vi "Init AI Resources.vi"(8 "error in (no error)":errorcluster, 11 "Session in":refnum<class "Session.lvclass">) -> (0 "error out":errorcluster, 3 "Session out":refnum<class "Session.lvclass">)   [LabVIEW 2024, in "CTI.lvlib" / "Session.lvclass"]
uses:
  Session.lvclass
  ADC Number.ctl
  AI/AI.lvclass
  Session.lvclass/Session.ctl
  CTI.lvlib
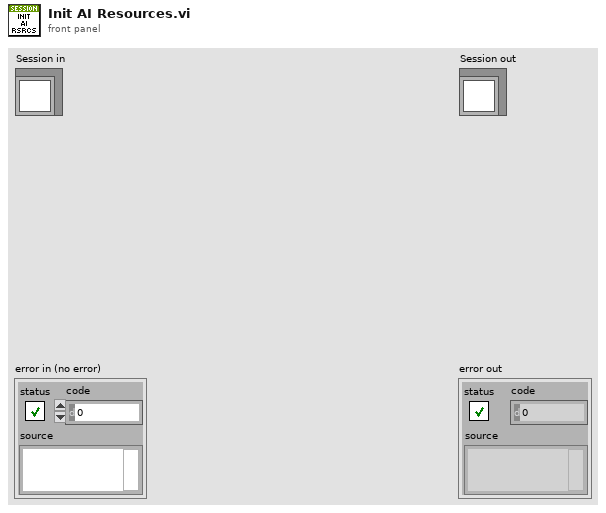
[diagram p1: front panel]
types:
  T1 = typedef "CTI.lvlib/ADC Number.ctl" = i8
  T2 = typedef "CTI.lvlib/Available AI.ctl" = cluster{"ADC #":T1, "GPIO #":T3}
  T3 = typedef "CTI.lvlib/GPIO Number.ctl" = i8
  T4 = typedef "CTI.lvlib/Session.lvclass/Resources.ctl" = cluster{"GPIO":map{T3, refnum<class "GPIO.lvclass">}, "AI":map{T1, refnum<class "AI.lvclass">}, "PWM":map{T3, refnum<class "PWM.lvclass">}, "UART":map{T5, refnum<class "UART.lvclass">}, "I2C":map{T6, refnum<class "I2C.lvclass">}, "SPI":map{T7, refnum<class "SPI.lvclass">}, "SPI CS":map{T3, refnum<class "SPI CS.lvclass">}}
  T5 = typedef "CTI.lvlib/UART Number.ctl" = i8
  T6 = typedef "CTI.lvlib/I2C Number.ctl" = i8
  T7 = typedef "CTI.lvlib/SPI Number.ctl" = i8
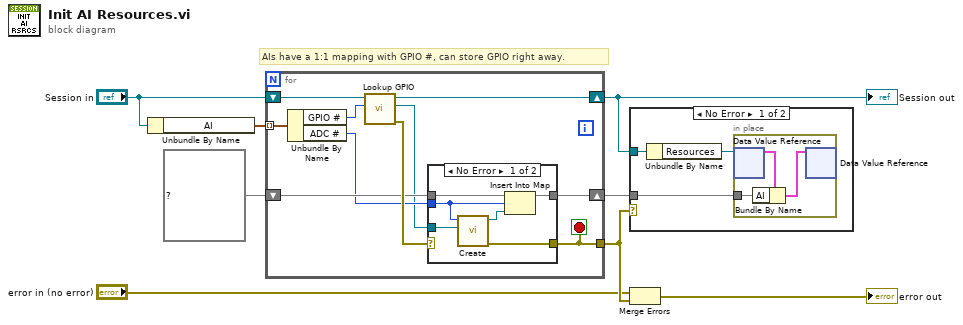
[diagram p0: block diagram]
diagram:
  # "AIs have a 1:1 mapping with GPIO #, can store GPIO right away."
  n1 = Unbundle By Name("Session in") -> ("AI"=w1:T2[])
  n2 = for {
    tunnel: w1 -> [w15] mode=indexing
    shift-right: [w16] -> w3
    shift-left: map{T1, refnum<class "AI.lvclass">} {} ("AI") -> [w17]
    shift-right: [w11] -> w8
    shift-left: "Session in" -> [w14]
    tunnel: [w9] -> w7
    stop <- w9 stop-if-true
    n3 = Unbundle By Name(w15) -> ("GPIO #"=w13:T3, "ADC #"=w12:T1)
    n4 = call "Lookup GPIO.vi"("GPIO #"=w13, "Session in"=w14) -> ("error out"=w18:errorcluster, "GPIO"=w10:refnum<class "GPIO.lvclass">, "Session out"=w11:refnum<class "Session.lvclass">)  [unwired: 7 in]
    n5 = case shown="No Error" w18 {
      selector: w18 -> [_ w26]
      tunnel: w17 -> [w24 w25]
      tunnel: [w23 w25] -> w16
      tunnel: w10 -> [w22 _]
      tunnel: w12 -> [w21 _]
      tunnel: [w19 w26] -> w9
      frame No Error {
        n6 = call "Create.vi"("GPIO"=w22, "ADC #"=w21) -> ("error out"=w19:errorcluster, "AnalogIn out"=w20:refnum<class "AI.lvclass">)  [unwired: 8 in]
        n7 = Insert Into Map(map in=w24, key=w21, value=w20) -> (map out=w23:map{T1, refnum<class "AI.lvclass">})  [unwired: 2 out]
      }
      frame Error {
      }
    }
  }
  "Session out" <- w8
  n8 = case shown="No Error" w7 {
    tunnel: w3 -> [w27 _]
    tunnel: w8 -> [w29 _]
    frame No Error {
      n9 = Unbundle By Name(w29) -> ("Resources"=w28:refnum<data-value>)
      n10 = in-place {
        in-place-border: w27 -> [w31]
        n11 = in-place-dvr #1(w28) -> (w32:T4)  [unwired: 1 out]
        n12 = Bundle By Name(cluster=w32, "AI"=w31) -> (w30:T4)
        n13 = in-place-dvr #1(w30) -> ()  [unwired: 2 out]
      }
    }
    frame Error {
    }
  }
  n14 = Merge Errors("error in (no error)", w7) -> (→"error out":errorcluster)
